vi "joystick scaleNtransform.vi"(9 "joystick values":dbl[](array[numeric])) -> (3 "Transformed joystick values":dbl[](array[numeric]))   [LabVIEW 2018]
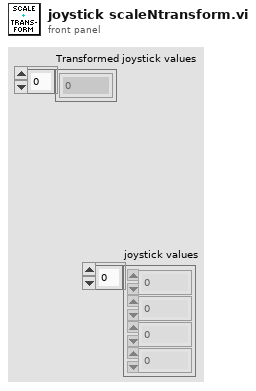
[diagram p1: front panel]
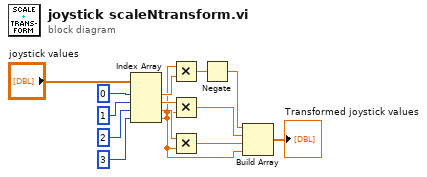
[diagram p0: block diagram]
diagram:
  n1 = Index Array(array="joystick values", index #1=0 ("index"), index #2=1 ("index"), index #3=2 ("index"), index #4=3 ("index")) -> (element #1=w9:dbl, element #2=w8:dbl, element #3=w7:dbl, element #4=w1:dbl)
  n2 = Multiply(x=w1, y=w9) -> (x*y=w6:dbl)
  n3 = Multiply(x=w8, y=w1) -> (x*y=w4:dbl)
  n4 = Multiply(x=w7, y=w1) -> (x*y=w2:dbl)
  n5 = Negate(x=w6) -> (-x=w5:dbl)
  n6 = Build Array(w5, w4, w2, w1) -> (→"Transformed joystick values":dbl[])
